vi "target.vi"() -> ()   [LabVIEW 2020]
uses:
  <vilib>/rvi/interface/RandomDataEmulation/niFpgaRandomDataHandleErrors.vi
  <vilib>/rvi/DataTransferAndStorage/Container/XNode/niFpgaContainer.xnode
  <vilib>/rvi/interface/RandomDataEmulation/nirviRandomDataFpgaReadWriteTemplate.vi
panel:
  out "Timed Out? FIFO in REAL":bool
  out "Timed Out? FIFO out index":bool
  out "Timed Out? FIFO out REAL":bool
  out "sort time (us)":u32
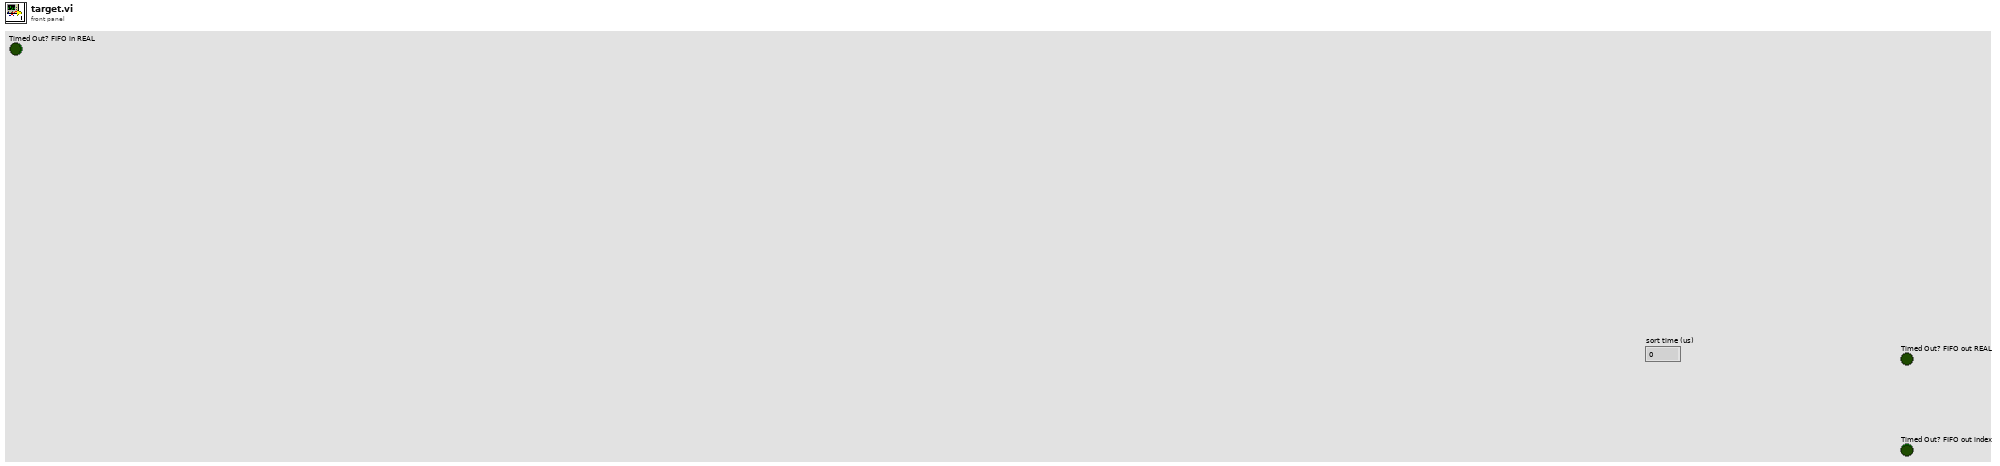
[diagram p1: front panel]
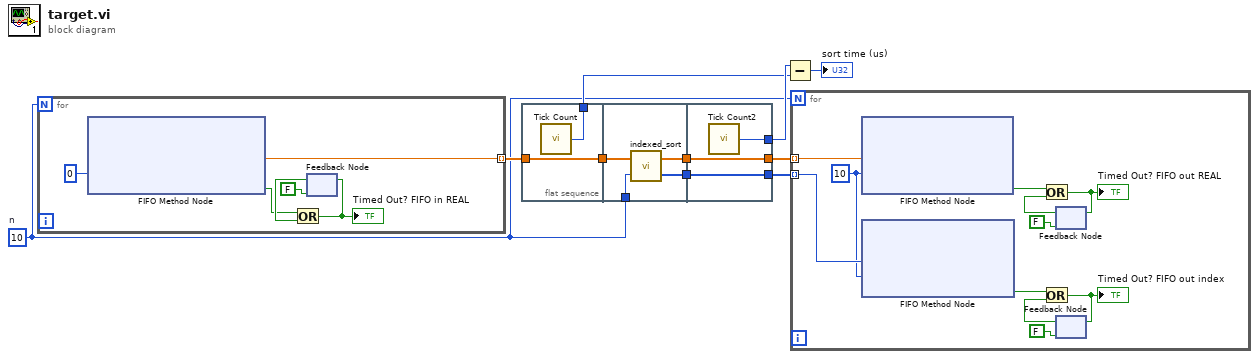
[diagram p0: block diagram]
diagram:
  w1 = 10  # n
  n1 = for {
    N: w1 -> [_]
    tunnel: [w11] -> w7 mode=indexing
    n2 = xnode ("FIFO Method Node")("Timeout"=0) -> ("Element"=w11:sgl, "Timed Out?"=w12:bool)  [unwired: 1 in, 1 out]
    n3 = feedback #1(FALSE) -> (w13:bool)
    n4 = Or(x=w12, y=w13) -> (x .or. y?=w14:bool)
    "Timed Out? FIFO in REAL" <- w14
    n5 = feedback-in #1(w14) -> ()
  }
  n6 = flat-sequence {
    tunnel: [w18] -> w9
    tunnel: w7 -> [w17]
    tunnel: [w17] -> w6
    tunnel: w1 -> [w22]
    tunnel: w6 -> [w19]
    tunnel: [w21] -> w5
    tunnel: [w20] -> w2
    tunnel: [w25] -> w10
    tunnel: [w24] -> w4
    tunnel: w5 -> [w24]
    tunnel: [w23] -> w3
    tunnel: w2 -> [w23]
    frame #0 {
      n7 = call "Tick Count"() -> ("Tick Count(uSec)"=w18:u32)
    }
    frame #1 {
      n8 = call "indexed_sort.vi"("n"=w22, "A"=w19) -> ("Index"=w20:i32[], "A Sorted"=w21:sgl[])
    }
    frame #2 {
      n9 = call "Tick Count2"() -> ("Tick Count(uSec)"=w25:u32)
    }
  }
  n10 = Subtract(x=w10, y=w9) -> (x-y=→"sort time (us)":u32)
  n11 = for {
    N: w1 -> [_]
    tunnel: w3 -> [w36] mode=indexing
    tunnel: w4 -> [w35] mode=indexing
    w34 = 10 ("Timeout")
    n12 = xnode ("FIFO Method Node")("Element"=w35, "Timeout"=w34) -> ("Timed Out?"=w30:bool)  [unwired: 1 in, 1 out]
    n13 = xnode ("FIFO Method Node")("Element"=w36, "Timeout"=w34) -> ("Timed Out?"=w26:bool)  [unwired: 1 in, 1 out]
    n14 = feedback #2(FALSE) -> (w31:bool)
    n15 = Or(x=w30, y=w31) -> (x .or. y?=w32:bool)
    "Timed Out? FIFO out REAL" <- w32
    n16 = feedback-in #2(w32) -> ()
    n17 = feedback #3(FALSE) -> (w29:bool)
    n18 = Or(x=w26, y=w29) -> (x .or. y?=w28:bool)
    "Timed Out? FIFO out index" <- w28
    n19 = feedback-in #3(w28) -> ()
  }
